vi "HRM-GUI_main.vi"(8 "error in (no error)":errorcluster, 11 "Init cluster":T1) -> (0 "error out":errorcluster)   [LabVIEW 2020]
uses:
  HRM-init_cluster.ctl
  HRM-User_events.ctl
panel:
  out "Pulse":dbl
  out "unfiltered wf":waveform(dbl)(graph)
  out "Filtered":waveform(dbl)(graph)
  in  "Addition signal to remove (0) [s]":dbl
  in  "Samples size (10) [s]":i32=10
  in  "Stop":bool
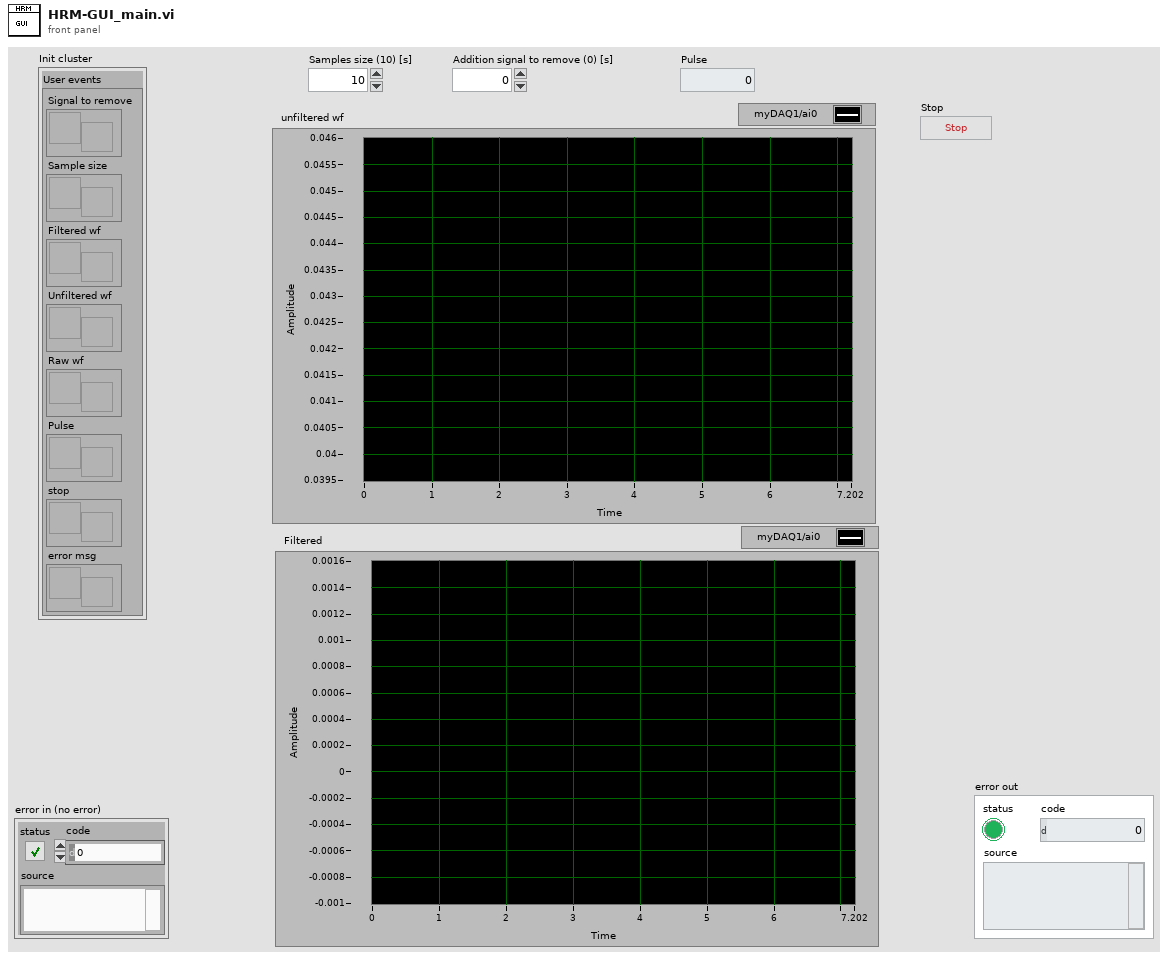
[diagram p1: front panel]
types:
  T1 = typedef "HRM-init_cluster.ctl" = cluster{"User events":T2}
  T2 = typedef "HRM-User_events.ctl" = cluster{"Signal to remove":refnum<user-event>, "Sample size":refnum<user-event>, "Filtered wf":refnum<user-event>, "Unfiltered wf":refnum<user-event>, "Raw wf":refnum<user-event>, "Pulse":refnum<user-event>, "stop":refnum<user-event>, "error msg":refnum<user-event>}
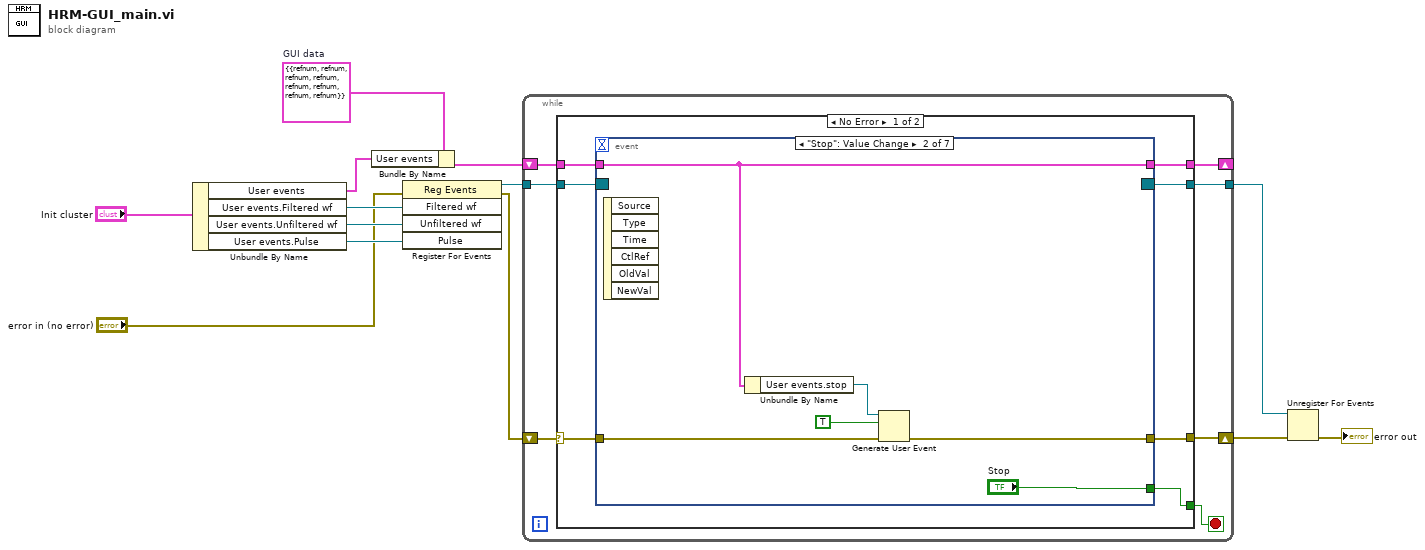
[diagram p0: block diagram]
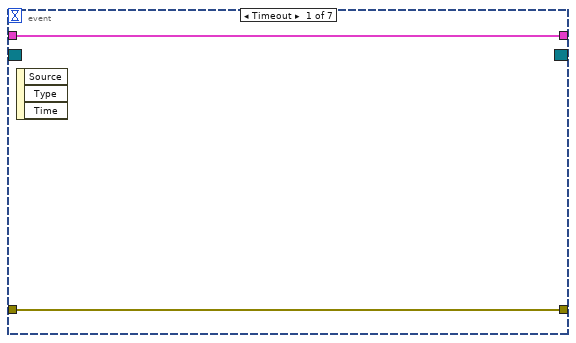
[diagram p2: hidden frame]
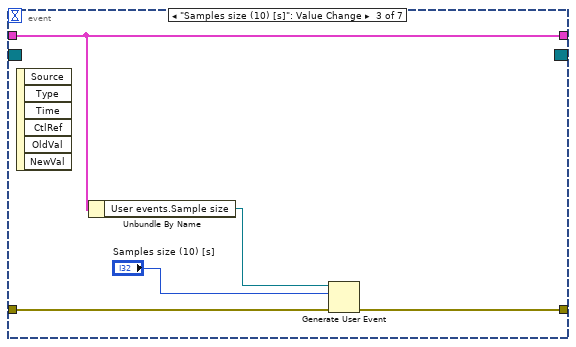
[diagram p3: hidden frame]
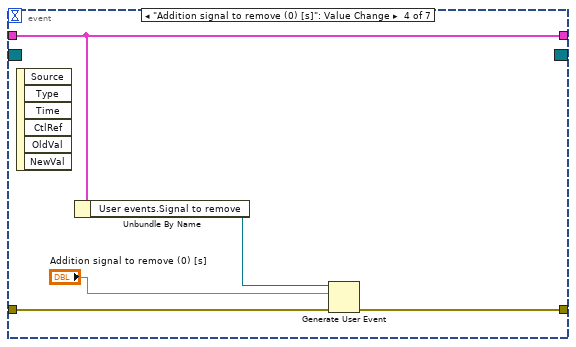
[diagram p4: hidden frame]
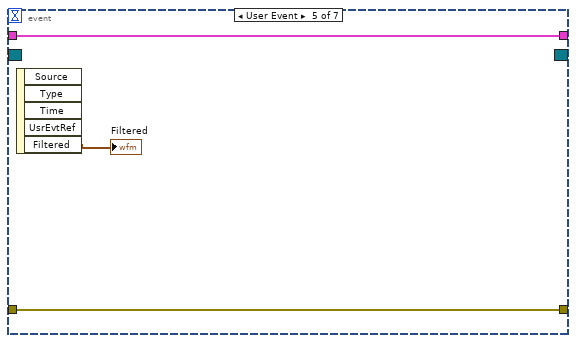
[diagram p5: hidden frame]
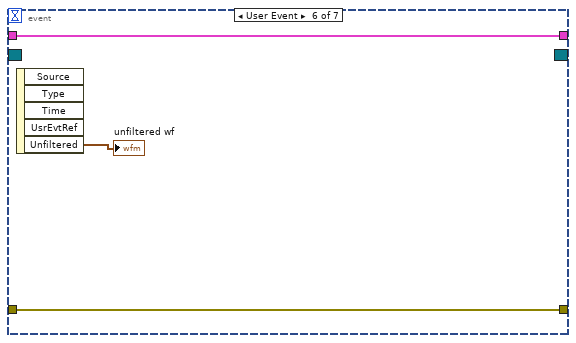
[diagram p6: hidden frame]
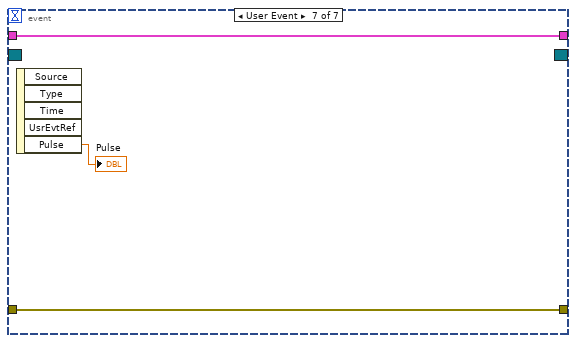
[diagram p7: hidden frame]
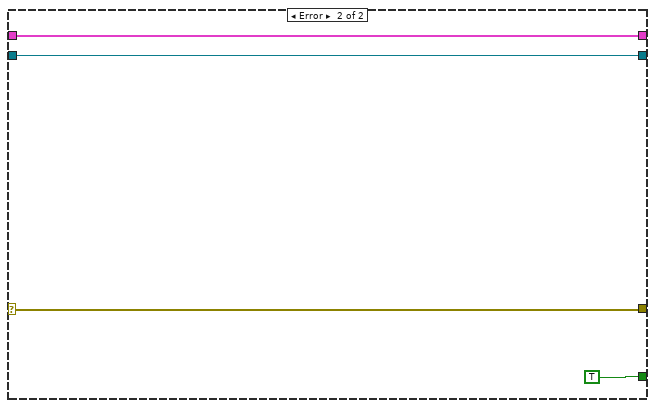
[diagram p8: hidden frame]
diagram:
  w12 = cluster{"User events":T2} {"User events"={"Signal to remove"=refnum, "Sample size"=refnum, "Filtered wf"=refnum, "Unfiltered wf"=refnum, "Raw wf"=refnum, "Pulse"=refnum, "stop"=refnum, "error msg"=refnum}}  # GUI data
  n1 = Unbundle By Name("Init cluster") -> ("User events"=w7:T2, "User events.Filtered wf"=w6:refnum<user-event>, "User events.Unfiltered wf"=w5:refnum<user-event>, "User events.Pulse"=w4:refnum<user-event>)
  n2 = Bundle By Name(cluster=w12, "User events"=w7) -> (w8:cluster{"User events":T2})
  n3 = register-events(error in="error in (no error)", w6, w5, w4) -> (reference out=w13:refnum<event-registration>, error out=w11:errorcluster)  [unwired: 1 in]
  n4 = while {
    tunnel: w13 -> [w20]
    shift-right: [w16] -> w9
    shift-left: w11 -> [w17]
    shift-right: [w15] -> _
    shift-left: w8 -> [w19]
    tunnel: [w14] -> w10
    stop <- w18 stop-if-true
    n5 = case shown="No Error" w17 {
      selector: w17 -> [w24 w57]
      tunnel: [w25 TRUE ("Stop")] -> w18
      tunnel: [w23 w57] -> w16
      tunnel: w20 -> [w27 w55]
      tunnel: w19 -> [w26 w56]
      tunnel: [w22 w56] -> w15
      tunnel: [w21 w55] -> w14
      frame No Error {
        n6 = event shown="[1] \"Stop\": Value Change" {
          selector: w27 -> [_ _ _ _ _ _ _]
          dyn-events: [_ _ _ _ _ _ _] -> w21
          timeout: _ -> [_ _ _ _ _ _ _]
          tunnel: w26 -> [w29 w34 w38 w43 w47 w50 w53]
          tunnel: [_ "Stop" _ _ _ _ _] -> w25
          tunnel: [w28 w31 w39 w44 w48 w51 w54] -> w23
          tunnel: w24 -> [w28 w32 w40 w45 w48 w51 w54]
          tunnel: [w29 w34 w38 w43 w47 w50 w53] -> w22
          event Timeout {
            n7 = event-data() -> ()  [unwired: 1 in, 3 out]
          }
          event "Stop": Value Change {
            n8 = event-data() -> ()  [unwired: 1 in, 6 out]
            n9 = Unbundle By Name(w34) -> ("User events.stop"=w33:refnum<user-event>)
            n10 = Generate User Event(user event=w33, event data cluster=TRUE ("event data"), error in=w32) -> (error out=w31:errorcluster)  [unwired: 1 in, 1 out]
          }
          event "Samples size (10) [s]": Value Change {
            n11 = event-data() -> ()  [unwired: 1 in, 6 out]
            n12 = Unbundle By Name(w38) -> ("User events.Sample size"=w37:refnum<user-event>)
            n13 = Generate User Event(user event=w37, event data cluster="Samples size (10) [s]", error in=w40) -> (error out=w39:errorcluster)  [unwired: 1 in, 1 out]
          }
          event "Addition signal to remove (0) [s]": Value Change {
            n14 = event-data() -> ()  [unwired: 1 in, 6 out]
            n15 = Unbundle By Name(w43) -> ("User events.Signal to remove"=w42:refnum<user-event>)
            n16 = Generate User Event(user event=w42, event data cluster="Addition signal to remove (0) [s]", error in=w45) -> (error out=w44:errorcluster)  [unwired: 1 in, 1 out]
          }
          event User Event {
            n17 = event-data() -> ("Filtered"=→"Filtered":waveform(dbl))  [unwired: 1 in, 4 out]
          }
          event User Event {
            n18 = event-data() -> ("Unfiltered"=→"unfiltered wf":waveform(dbl))  [unwired: 1 in, 4 out]
          }
          event User Event {
            n19 = event-data() -> ("Pulse"=→"Pulse":dbl)  [unwired: 1 in, 4 out]
          }
        }
      }
      frame Error {
      }
    }
  }
  n20 = Unregister For Events(event registration refnum=w10, error in=w9) -> (error out=→"error out":errorcluster)
